vi "Main FPGA 8-axis_4.vi"() -> ()   [LabVIEW 2014]
uses:
  <vilib>/Motion/MotorControl/_s/nism.interpretControlRegister.stateTransition.ctl
  <vilib>/Platform/TimedLoop/XDataNode/timing_clust.ctl
  <vilib>/Platform/TimedLoop/XDataNode/nitl_modes.ctl
  <vilib>/Platform/TimedLoop/XDataNode/wakeup.ctl
  <vilib>/rvi/Emulation/niFpgaGetClockAttributes.vi
  <vilib>/rvi/Emulation/niFpgaSctlEmulationGetInTimedLoop.vi
  <vilib>/rvi/Emulation/niFpgaEmulationReportErrorSimple.vi
  Global FPGA 8-axis.vi
  <vilib>/rvi/eio/common/nirviEmuTemplateMethod_errors.vi
  <vilib>/Motion/MotorControl/_s/nism.interpretControlRegister.indexed.vi
  <vilib>/rvi/Emulation/niFpgaProcessEmulError.vi
  <vilib>/Motion/MotorControl/_s/nism.mdo.read.positionLoopSyncData.vi
  <vilib>/Motion/MotorControl/_s/nism.mdo.read.splineData.vi
  <vilib>/Motion/MotorControl/_s/nism.generateStatusRegister.indexed.vi
  <vilib>/rvi/Emulation/niFpgaCriticalErrorInLSC.vi
  <vilib>/Motion/MotorControl/_s/nism.splineInterpolation.fxp.3.index.vi
  <vilib>/Motion/MotorControl/_s/nism.mdo.handler.indexed.vi
  <vilib>/Motion/SoftMotion/Synchronization/nism.rioScan.generateSyncScan.vi
  <vilib>/eio/EIONode/EIONode.xnode
  <vilib>/Platform/TimedLoop/XDataNode/XDataNode.xnode
  <vilib>/Motion/MotorControl/NI_SoftMotion_MotorControlIP.lvlib
  <vilib>/Platform/TimedLoop/XDataNode/XDNodeRunTimeDep.lvlib
  <vilib>/Motion/SoftMotion/Synchronization/NI_SoftMotion_Synchronization.lvlib
panel:
  out "Interpolated Positions":fxp<+/-,64,32>[](array[numeric])
  in  "minimum pulse":u16=40
  in  "Invert direction?":bool
  in  "Enable Drives?":bool
  out "State":T1=enum."Start --> Initializing" caption="state transition"
  in  "Sync Value":bool
  in  "Sync Enable override?":bool
  out "Sync is Fault":bool
  out "Sync is Locked":bool
  # "Synchronization Loop"
  # "Control Status Loop"
  # "Notes: \n1. This VI provides the communication interface between the NI SoftMotion Engine and the LabVIEW FPGA Module. You must compile this VI for a specific FPGA target before use. After compiling, run the VI before running any of the Express VI examples. For information on moving this example to another FPGA target, refer to ni.com/info and enter info code fpgaex.\n\n2. Only use the Reset Axis button if you are unable to communicate with the axis by any other means. This button resets the device state machine and other VIs to a known state. After resetting the axis, switch the NI Scan Engine from Active Mode to Configuration Mode, then back to Active Mode, before attempting to enable the axis."
  # "(These two buttons \nare for testing\npurposes.)"
  # "Step/Direction Loop"
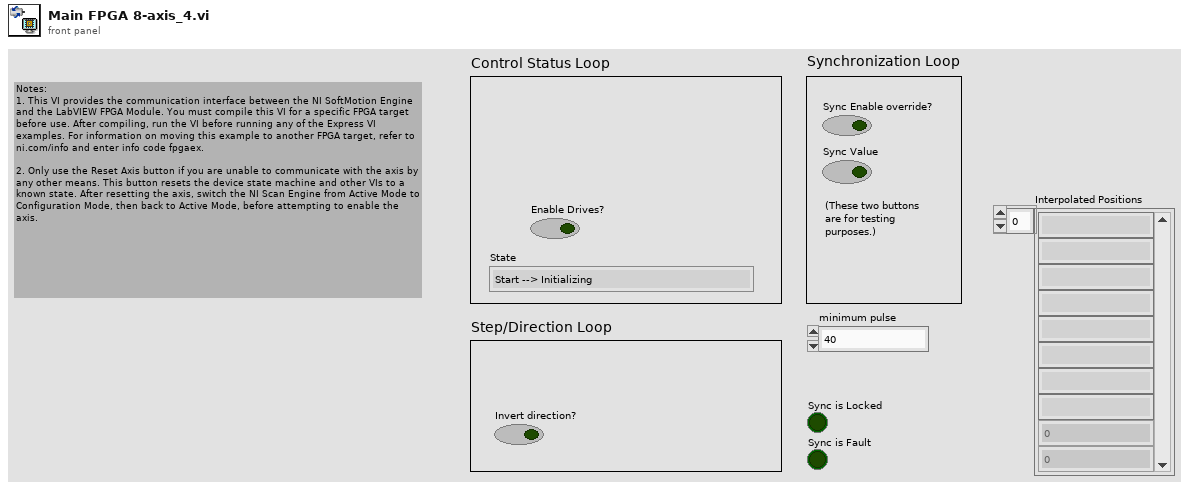
[diagram p1: front panel]
types:
  T1 = typedef "NI_SoftMotion_MotorControlIP.lvlib/nism.interpretControlRegister.stateTransition.ctl" = enum8{"Invalid", "Start --> Initializing", "Initializing --> Disabled", "Disabled --> Ready To Switch On", "Ready To Switch On --> Switched On", "Ready To Switch On --> Disable", "Switched On --> Operation Enable", "Switched On --> Ready To Switch On", "Switched On --> Disabled", "Operation Enable --> Switched On", "Operation Enable --> Ready To Switch On", "Operation Enable --> Disabled", "Fault --> Disabled", "Any --> Fault", "None"}
  T2 = typedef "NI_SoftMotion_MotorControlIP.lvlib/nism.mdo.splineData.ctl" = cluster{"spline type":T3, "traj per/spline per":u16, "spline per/traj per":fxp<+,32,0>}
  T3 = typedef "NI_SoftMotion_MotorControlIP.lvlib/nism.splineInterpolation.type.ctl" = u16
  T4 = typedef "NI_SoftMotion_Synchronization.lvlib/nism.softmotionScan.timerConfig.ctl" = cluster{"target period (clocks)":u16, "host period / target period":u16}
  T5 = typedef "NI_SoftMotion_Synchronization.lvlib/nism.softmotionScan.timerControl.ctl" = cluster{"sm scan":bool, "sm scan count":u32, "sm scan enabled":bool}
  T6 = typedef "XDNodeRunTimeDep.lvlib/timing_clust.ctl" = cluster{"Expected End [f-1]":u64, "Actual End [f-1]":u64, "Finished Late? [f-1]":bool, "Expected End [i-1]":u64, "Actual End [i-1]":u64, "Finished Late? [i-1]":bool, "Expected Start [i]":u64, "Actual Start [i]":u64, "Expected Start [f]":u64, "Actual Start [f]":u64, "Source Name":string, "Structure Name":string, "Period":i64, "Deadline":i64, "Offset":i64, "Start":i64, "Priority":i32, "Timeout":i32, "Mode":T7, "Wakeup Reason":T8, "Error":errorcluster, "Source Type":string, "Secondary Source Type":string, "Global End Time":u64, "Global Start Time":u64, "Frame Duration":u64, "Iteration Duration":u64, "Assigned CPU":i32, "I/O Scan Engine Mode":u32}
  T7 = typedef "XDNodeRunTimeDep.lvlib/nitl_modes.ctl" = enum32{"No Change", "Process missed periods, maintain original phase", "Discard missed periods, maintain original phase", "Process missed periods, ignore original phase", "Discard missed periods, ignore original phase"}
  T8 = typedef "XDNodeRunTimeDep.lvlib/wakeup.ctl" = enum32{"Normal", "Aborted", "Asynchronous wakeup", "Timing source error", "Timed loop error", "Timeout"}
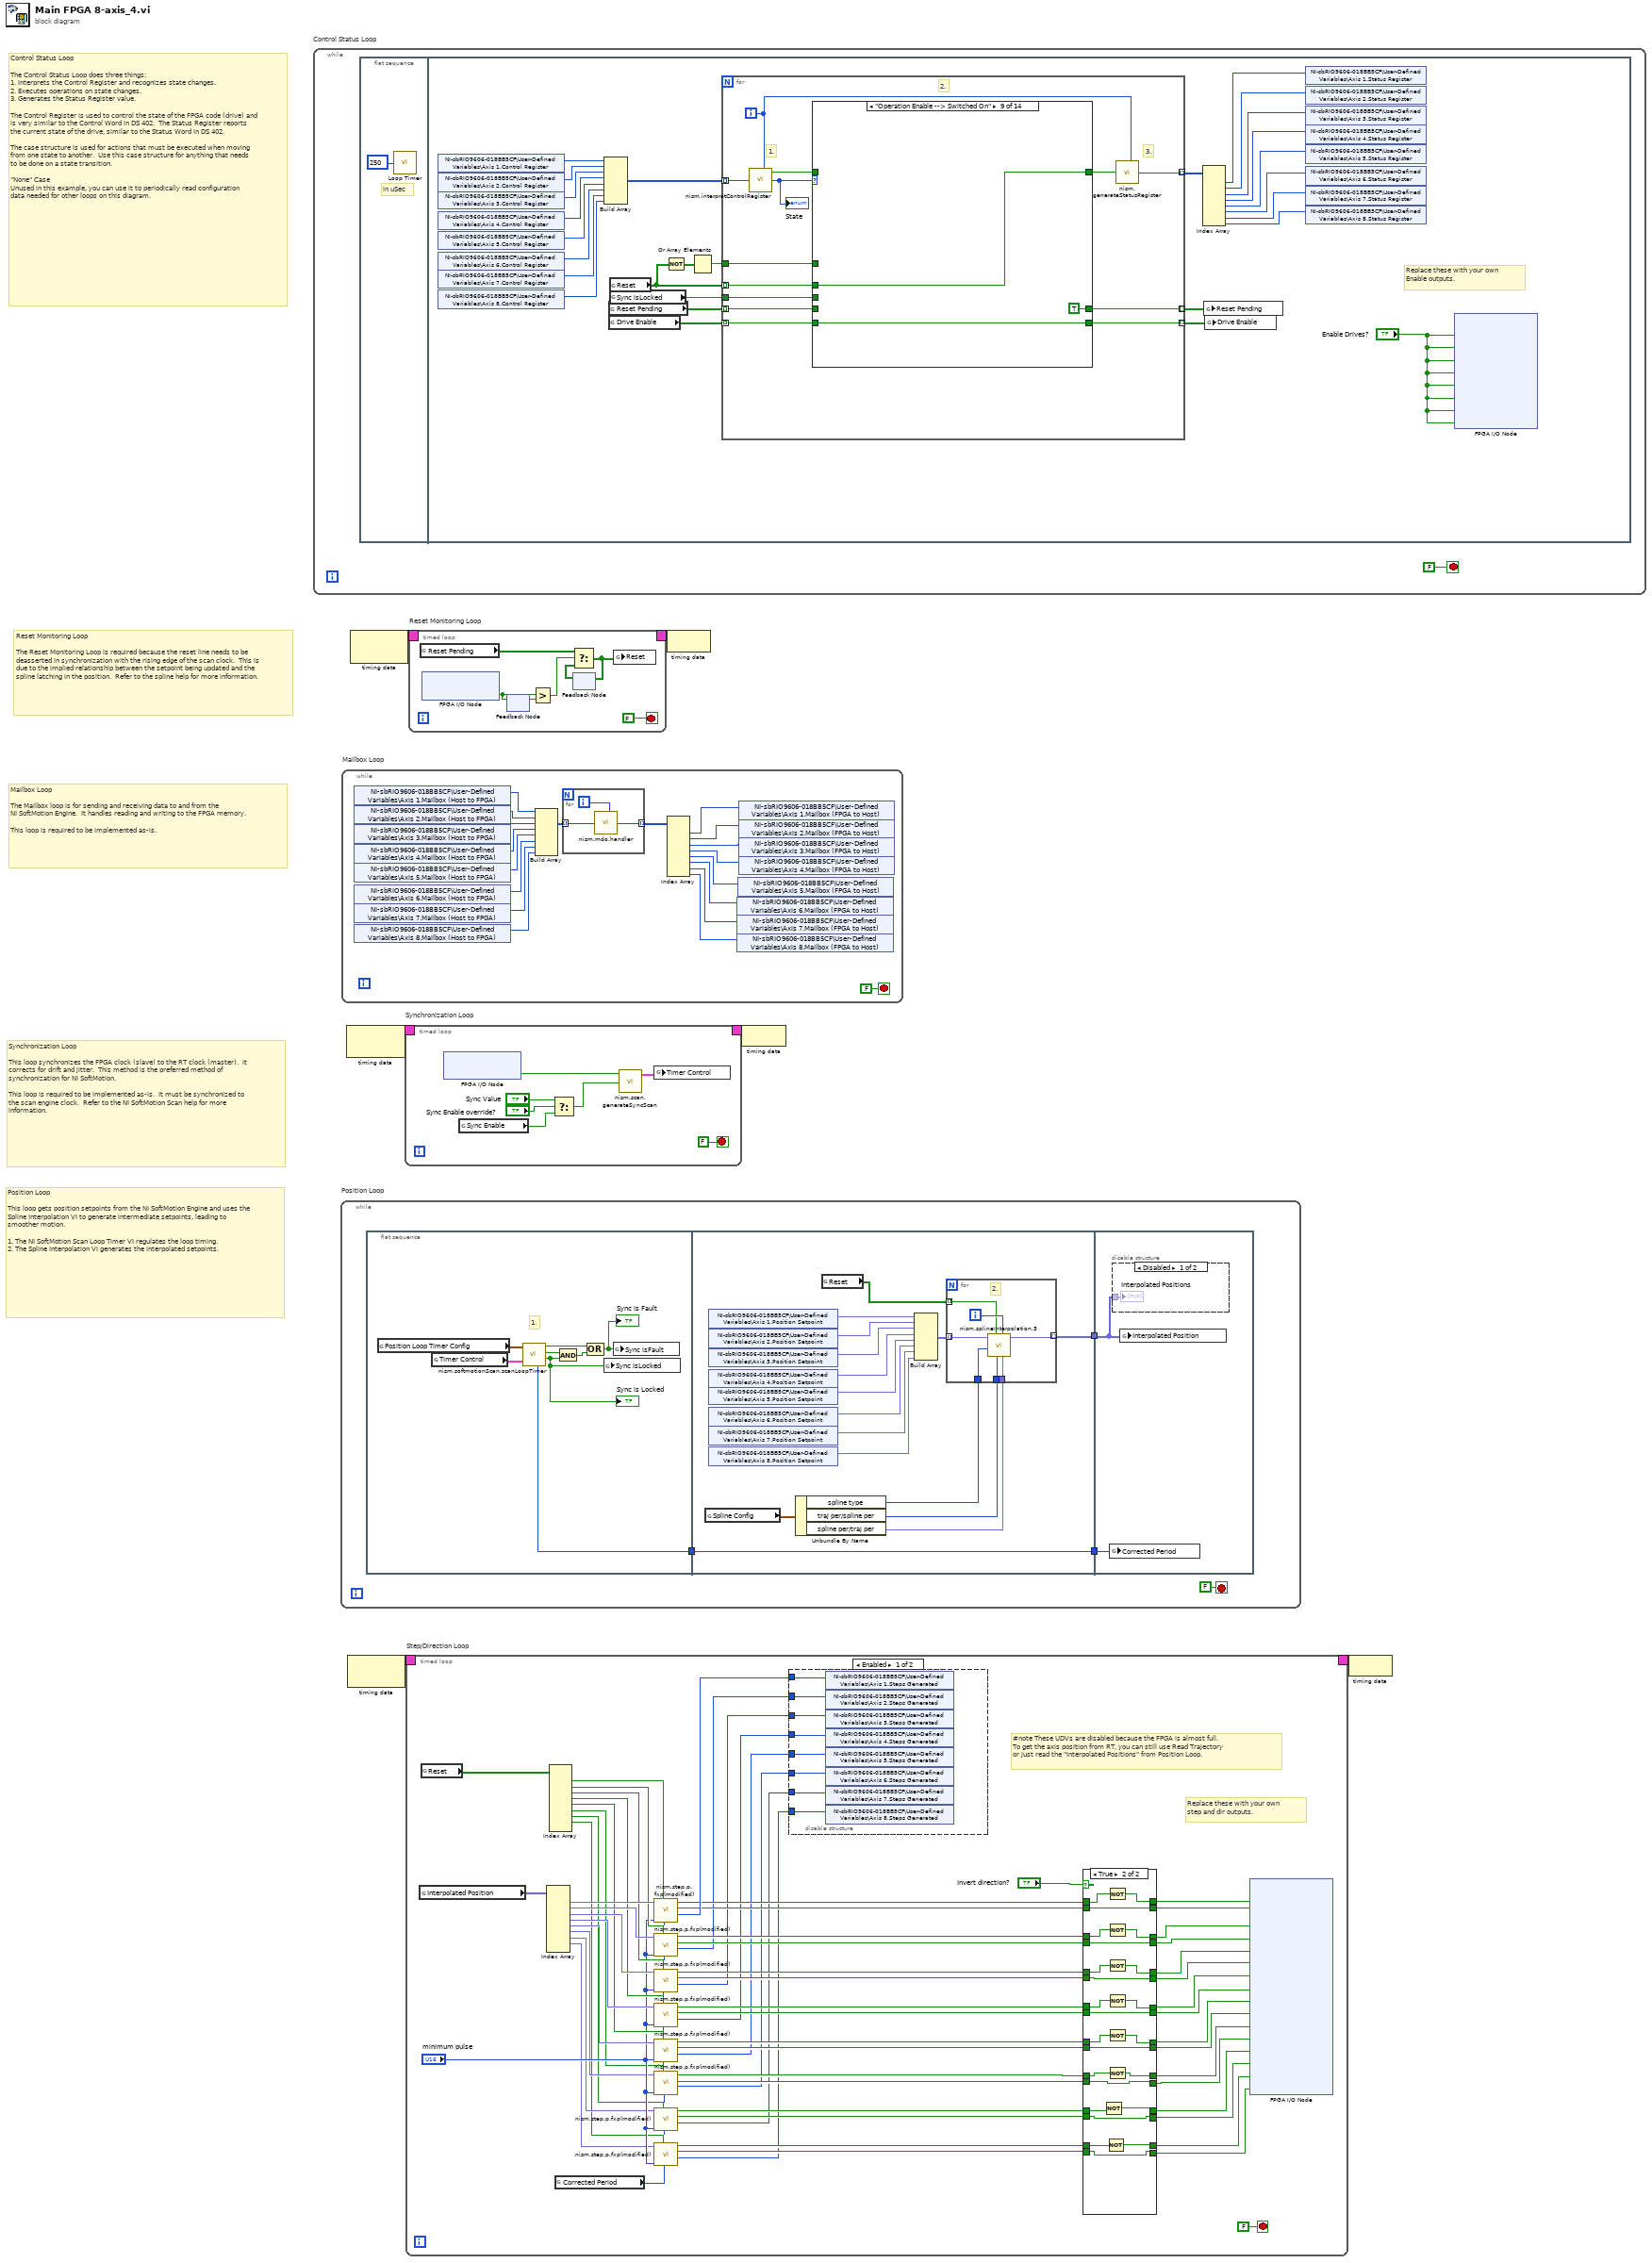
[diagram p0: block diagram]
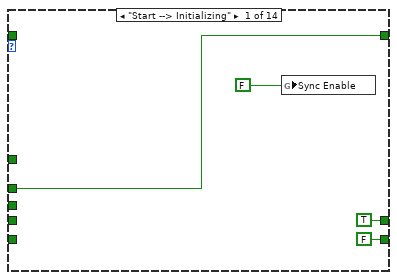
[diagram p5: hidden frame]
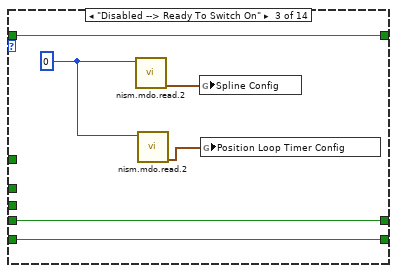
[diagram p7: hidden frame]
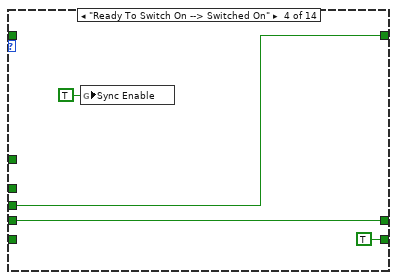
[diagram p8: hidden frame]
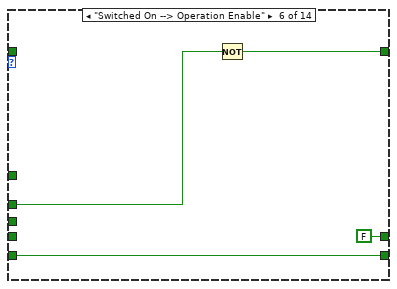
[diagram p10: hidden frame]
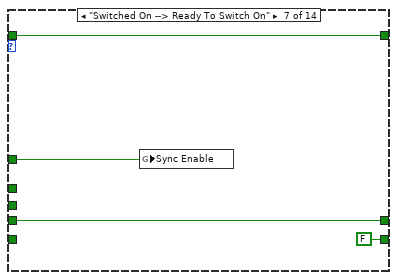
[diagram p11: hidden frame]
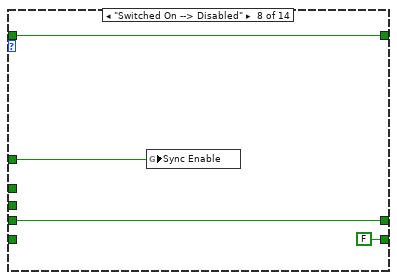
[diagram p12: hidden frame]
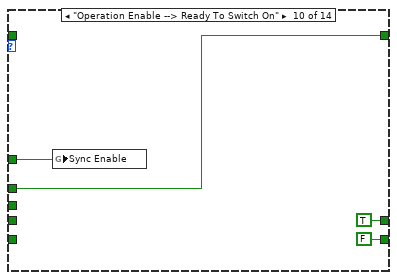
[diagram p13: hidden frame]
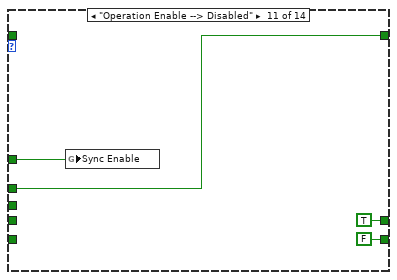
[diagram p14: hidden frame]
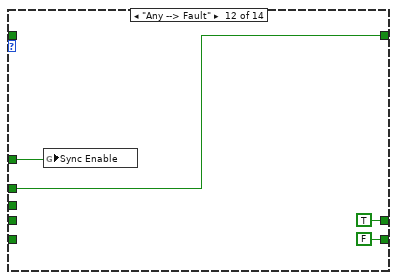
[diagram p15: hidden frame]
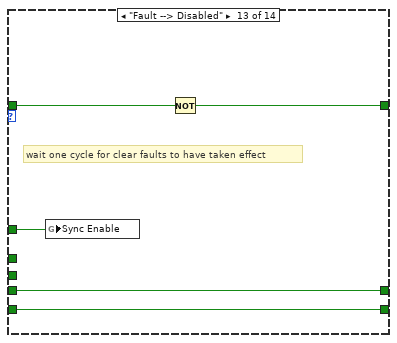
[diagram p16: hidden frame]
diagram:
  # "Position Loop\n\nThis loop gets position setpoints from the NI SoftMotion Engine and uses the Spline Interpolation VI to generate intermediate setpoints, leading to smoother motion.\n\n1. The NI SoftMotion Scan Loop Timer VI regulates the loop timing. \n2. The Spline Interpolation VI generates the interpolated setpoints."
  # "Synchronization Loop\n\nThis loop synchronizes the FPGA clock (slave) to the RT clock (master).  It corrects for drift and jitter.  This method is the preferred method of synchronization for NI SoftMotion.\n\nThis loop is required to be implemented as-is.  It must be synchronized to the scan engine clock.  Refer to the NI SoftMotion Scan help for more information."
  # "Mailbox Loop\n\nThe Mailbox loop is for sending and receiving data to and from the \nNI SoftMotion Engine.  It handles reading and writing to the FPGA memory.\n\nThis loop is required to be implemented as-is."
  # "Reset Monitoring Loop\n\nThe Reset Monitoring Loop is required because the reset line needs to be deasserted in synchronization with the rising edge of the scan clock.  This is due to the implied relationship between the setpoint being updated and the spline latching in the position.  Refer to the spline help for more information."
  # "Control Status Loop\n\nThe Control Status Loop does three things:\n1. Interprets the Control Register and recognizes state changes.\n2. Executes operations on state changes.\n3. Generates the Status Register value.\n\nThe Control Register is used to control the state of the FPGA code (drive) and is very similar to the Control Word in DS 402.  The Status Register reports the current state of the drive, similar to the Status Word in DS 402.\n\nThe case structure is used for actions that must be executed when moving from one state to another.  Use this case structure for anything that needs to be done on a state transition.\n\n\"None\" Case\nUnused in this example, you can use it to periodically read configuration data needed for other loops on this diagram."
  n1 = while "Control Status Loop" {
    stop <- FALSE stop-if-true
    n2 = flat-sequence {
      frame #0 {
        # "in uSec"
        n3 = call "Loop Timer"("Count(uSec)"=u32 250) -> ()  [unwired: 1 out]
      }
      frame #1 {
        # "Replace these with your own\nEnable outputs."
        n4 = shared-variable "NI-sbRIO9606-018BB5CF\\User-Defined Variables\\Axis 1.Control Register"() -> (w25:u32)  [unwired: 1 in, 1 out]
        n5 = shared-variable "NI-sbRIO9606-018BB5CF\\User-Defined Variables\\Axis 2.Control Register"() -> (w24:u32)  [unwired: 1 in, 1 out]
        n6 = shared-variable "NI-sbRIO9606-018BB5CF\\User-Defined Variables\\Axis 3.Control Register"() -> (w23:u32)  [unwired: 1 in, 1 out]
        n7 = shared-variable "NI-sbRIO9606-018BB5CF\\User-Defined Variables\\Axis 4.Control Register"() -> (w22:u32)  [unwired: 1 in, 1 out]
        n8 = shared-variable "NI-sbRIO9606-018BB5CF\\User-Defined Variables\\Axis 5.Control Register"() -> (w21:u32)  [unwired: 1 in, 1 out]
        n9 = shared-variable "NI-sbRIO9606-018BB5CF\\User-Defined Variables\\Axis 6.Control Register"() -> (w15:u32)  [unwired: 1 in, 1 out]
        n10 = shared-variable "NI-sbRIO9606-018BB5CF\\User-Defined Variables\\Axis 7.Control Register"() -> (w14:u32)  [unwired: 1 in, 1 out]
        n11 = shared-variable "NI-sbRIO9606-018BB5CF\\User-Defined Variables\\Axis 8.Control Register"() -> (w13:u32)  [unwired: 1 in, 1 out]
        n12 = Build Array(w25, w24, w23, w22, w21, w15, w14, w13) -> (w34:u32[])
        n13 = global read "Global FPGA 8-axis.vi" "Reset Pending"() -> (w29:bool[])
        n14 = global read "Global FPGA 8-axis.vi" "Drive Enable"() -> (w28:bool[])
        n15 = global read "Global FPGA 8-axis.vi" "Reset"() -> (w30:bool[])
        n16 = global read "Global FPGA 8-axis.vi" "Sync isLocked"() -> (w35:bool)
        n17 = Not(x=w30) -> (.not. x?=w32:bool[])
        n18 = Or Array Elements(Boolean array=w32) -> (logical OR=w31:bool)
        n19 = for {
          tunnel: w30 -> [w43] mode=indexing
          tunnel: w35 -> [w42]
          tunnel: w34 -> [w44] mode=indexing
          tunnel: [w41] -> w26 mode=indexing
          tunnel: [w40] -> w33 mode=indexing
          tunnel: [w39] -> w27 mode=indexing
          tunnel: w31 -> [w38]
          tunnel: w29 -> [w37] mode=indexing
          tunnel: w28 -> [w36] mode=indexing
          i -> [w45]
          # "3."
          # "2."
          # "1."
          n20 = call-poly <vilib>:"nism.interpretControlRegister.vi"("control register"=w44, "axis index"=w45) -> ("transition occurred"=w46:bool, "state transition"=w47:T1)  [unwired: 6 in]
          "State" <- w47
          n21 = case shown="\"Operation Enable --> Switched On\"" w47 {
            tunnel: w46 -> [_ w55 w61 _ w68 _ w76 w80 _ _ _ _ w100 _]
            tunnel: [w52 w55 w61 w63 w68 w72 w76 w80 w82 w85 w89 w93 w99 _] -> w48
            tunnel: w43 -> [w52 _ _ _ _ w71 _ _ w82 w85 w89 w93 _ _]
            tunnel: w42 -> [_ _ _ w63 _ _ _ _ _ _ _ _ _ _]
            tunnel: [TRUE ("Write.Reset Pending") w54 w57 w62 w67 FALSE ("Write.Reset Pending") w73 w77 TRUE ("Write.Reset Pending") TRUE ("Write.Reset Pending") TRUE ("Write.Reset Pending") TRUE ("Write.Reset Pending") w97 w102] -> w40
            tunnel: [FALSE ("Write.Drive Enable") w53 w56 TRUE ("Write.Drive Enable") w66 w69 FALSE ("Write.Drive Enable") FALSE ("Write.Drive Enable") w81 FALSE ("Write.Drive Enable") FALSE ("Write.Drive Enable") FALSE ("Write.Drive Enable") w96 w101] -> w39
            tunnel: w38 -> [_ _ _ _ _ _ w74 w78 _ w84 w88 w92 w98 _]
            tunnel: w37 -> [_ w54 w57 w62 w67 _ w73 w77 _ _ _ _ w97 w102]
            tunnel: w36 -> [_ w53 w56 _ w66 w69 _ _ w81 _ _ _ w96 w101]
            frame "Start --> Initializing" {
              n22 = global write "Global FPGA 8-axis.vi" "Sync Enable"(FALSE ("Sync Enable")) -> ()
            }
            frame "Initializing --> Disabled" {
            }
            frame "Disabled --> Ready To Switch On" {
              w59 = 0 ("axis index")
              n23 = call-poly <vilib>:"nism.mdo.read.2.vi"("axis index"=w59) -> ("spline"=w60:T2)  [unwired: 10 in]
              n24 = call-poly <vilib>:"nism.mdo.read.2.vi"("axis index"=w59) -> ("position loop sync"=w58:T4)  [unwired: 10 in]
              n25 = global write "Global FPGA 8-axis.vi" "Spline Config"(w60) -> ()
              n26 = global write "Global FPGA 8-axis.vi" "Position Loop Timer Config"(w58) -> ()
            }
            frame "Ready To Switch On --> Switched On" {
              n27 = global write "Global FPGA 8-axis.vi" "Sync Enable"(TRUE ("Sync Enable")) -> ()
            }
            frame "Ready To Switch On --> Disable" {
            }
            frame "Switched On --> Operation Enable" {
              n28 = Not(x=w71) -> (.not. x?=w72:bool)
            }
            frame "Switched On --> Ready To Switch On" {
              n29 = global write "Global FPGA 8-axis.vi" "Sync Enable"(w74) -> ()
            }
            frame "Switched On --> Disabled" {
              n30 = global write "Global FPGA 8-axis.vi" "Sync Enable"(w78) -> ()
            }
            frame "Operation Enable --> Switched On" {
            }
            frame "Operation Enable --> Ready To Switch On" {
              n31 = global write "Global FPGA 8-axis.vi" "Sync Enable"(w84) -> ()
            }
            frame "Operation Enable --> Disabled" {
              n32 = global write "Global FPGA 8-axis.vi" "Sync Enable"(w88) -> ()
            }
            frame "Any --> Fault" {
              n33 = global write "Global FPGA 8-axis.vi" "Sync Enable"(w92) -> ()
            }
            frame "Fault --> Disabled" {
              # "wait one cycle for clear faults to have taken effect"
              n34 = global write "Global FPGA 8-axis.vi" "Sync Enable"(w98) -> ()
              n35 = Not(x=w100) -> (.not. x?=w99:bool)
            }
            frame "None", Default {
            }
          }
          n36 = call-poly <vilib>:"nism.generateStatusRegister.vi"("transition success"=w48, "axis index"=w45) -> ("status register"=w41:u32)  [unwired: 7 in]
        }
        n37 = Index Array(array=w26) -> (element #1=w20:u32, element #2=w19:u32, element #3=w18:u32, element #4=w17:u32, element #5=w16:u32, element #6=w12:u32, element #7=w11:u32, element #8=w10:u32)  [unwired: 8 in]
        n38 = global write "Global FPGA 8-axis.vi" "Reset Pending"(w33) -> ()
        n39 = global write "Global FPGA 8-axis.vi" "Drive Enable"(w27) -> ()
        n40 = shared-variable "NI-sbRIO9606-018BB5CF\\User-Defined Variables\\Axis 1.Status Register"(w20) -> ()  [unwired: 1 in, 1 out]
        n41 = shared-variable "NI-sbRIO9606-018BB5CF\\User-Defined Variables\\Axis 2.Status Register"(w19) -> ()  [unwired: 1 in, 1 out]
        n42 = shared-variable "NI-sbRIO9606-018BB5CF\\User-Defined Variables\\Axis 3.Status Register"(w18) -> ()  [unwired: 1 in, 1 out]
        n43 = shared-variable "NI-sbRIO9606-018BB5CF\\User-Defined Variables\\Axis 4.Status Register"(w17) -> ()  [unwired: 1 in, 1 out]
        n44 = shared-variable "NI-sbRIO9606-018BB5CF\\User-Defined Variables\\Axis 5.Status Register"(w16) -> ()  [unwired: 1 in, 1 out]
        n45 = shared-variable "NI-sbRIO9606-018BB5CF\\User-Defined Variables\\Axis 6.Status Register"(w12) -> ()  [unwired: 1 in, 1 out]
        n46 = shared-variable "NI-sbRIO9606-018BB5CF\\User-Defined Variables\\Axis 7.Status Register"(w11) -> ()  [unwired: 1 in, 1 out]
        n47 = shared-variable "NI-sbRIO9606-018BB5CF\\User-Defined Variables\\Axis 8.Status Register"(w10) -> ()  [unwired: 1 in, 1 out]
        n48 = xnode "FPGA I/O Node"("RMC/DIO15"="Enable Drives?", "RMC/DIO79"="Enable Drives?", "RMC/DIO78"="Enable Drives?", "RMC/DIO13"="Enable Drives?", "RMC/DIO62"="Enable Drives?", "RMC/DIO61"="Enable Drives?", "RMC/DIO76"="Enable Drives?", "RMC/DIO11"="Enable Drives?") -> ()  [unwired: 8 in, 8 out]
      }
    }
  }
  n49 = while "Position Loop" {
    stop <- FALSE stop-if-true
    n50 = flat-sequence {
      tunnel: [w107] -> w103
      tunnel: [w124] -> w105
      tunnel: [w123] -> w104
      tunnel: w103 -> [w123]
      tunnel: w105 -> [w138]
      tunnel: w104 -> [w139]
      frame #0 {
        # "1."
        n51 = global read "Global FPGA 8-axis.vi" "Position Loop Timer Config"() -> (w109:T4)
        n52 = global read "Global FPGA 8-axis.vi" "Timer Control"() -> (w108:T5)
        n53 = call <vilib>:"nism.softmotionScan.scanLoopTimer.vi"("timer control"=w108, "timer config"=w109) -> ("scan running?"=w111:bool, "finished late?"=w113:bool, "fault occurred?"=w114:bool, "corrected period"=w107:u16)  [unwired: 5 in, 1 out]
        "Sync is Locked" <- w111
        n54 = Compound Arithmetic op=AND(w113, w111) -> (w112:bool)
        n55 = Compound Arithmetic op=OR(w114, w112) -> (w110:bool)
        "Sync is Fault" <- w110
        n56 = global write "Global FPGA 8-axis.vi" "Sync isLocked"(w111) -> ()
        n57 = global write "Global FPGA 8-axis.vi" "Sync isFault"(w110) -> ()
      }
      frame #1 {
        n58 = global read "Global FPGA 8-axis.vi" "Spline Config"() -> (w126:T2)
        n59 = shared-variable "NI-sbRIO9606-018BB5CF\\User-Defined Variables\\Axis 1.Position Setpoint"() -> (w122:fxp<+/-,64,32>)  [unwired: 1 in, 1 out]
        n60 = shared-variable "NI-sbRIO9606-018BB5CF\\User-Defined Variables\\Axis 2.Position Setpoint"() -> (w121:fxp<+/-,64,32>)  [unwired: 1 in, 1 out]
        n61 = shared-variable "NI-sbRIO9606-018BB5CF\\User-Defined Variables\\Axis 3.Position Setpoint"() -> (w120:fxp<+/-,64,32>)  [unwired: 1 in, 1 out]
        n62 = shared-variable "NI-sbRIO9606-018BB5CF\\User-Defined Variables\\Axis 4.Position Setpoint"() -> (w119:fxp<+/-,64,32>)  [unwired: 1 in, 1 out]
        n63 = shared-variable "NI-sbRIO9606-018BB5CF\\User-Defined Variables\\Axis 5.Position Setpoint"() -> (w118:fxp<+/-,64,32>)  [unwired: 1 in, 1 out]
        n64 = shared-variable "NI-sbRIO9606-018BB5CF\\User-Defined Variables\\Axis 6.Position Setpoint"() -> (w117:fxp<+/-,64,32>)  [unwired: 1 in, 1 out]
        n65 = shared-variable "NI-sbRIO9606-018BB5CF\\User-Defined Variables\\Axis 7.Position Setpoint"() -> (w116:fxp<+/-,64,32>)  [unwired: 1 in, 1 out]
        n66 = shared-variable "NI-sbRIO9606-018BB5CF\\User-Defined Variables\\Axis 8.Position Setpoint"() -> (w115:fxp<+/-,64,32>)  [unwired: 1 in, 1 out]
        n67 = Unbundle By Name(w126) -> ("spline type"=w130:T3, "traj per/spline per"=w129:u16, "spline per/traj per"=w128:fxp<+,32,0>)
        n68 = global read "Global FPGA 8-axis.vi" "Reset"() -> (w125:bool[])
        n69 = Build Array(w122, w121, w120, w119, w118, w117, w116, w115) -> (w127:fxp<+/-,64,32>[])
        n70 = for {
          tunnel: w130 -> [w137]
          tunnel: w129 -> [w136]
          tunnel: w128 -> [w135]
          tunnel: w125 -> [w132] mode=indexing
          tunnel: w127 -> [w134] mode=indexing
          tunnel: [w131] -> w124 mode=indexing
          i -> [w133]
          # "2."
          n71 = call-poly <vilib>:"nism.splineInterpolation.3.vi"("1 / calls per sample"=w135, "index"=w133, "calls per sample"=w136, "reset"=w132, "spline type"=w137, "x"=w134) -> ("xi"=w131:fxp<+/-,64,32>)  [unwired: 4 in, 1 out]
        }
      }
      frame #2 {
        n72 = global write "Global FPGA 8-axis.vi" "Corrected Period"(w139) -> ()
        n73 = disable-structure shown="Disabled" {
          disable-tunnel: w138 -> [w140 _]
          frame Disabled {
            "Interpolated Positions" <- w140
          }
          frame Enabled {
          }
        }
        n74 = global write "Global FPGA 8-axis.vi" "Interpolated Position"(w138) -> ()
      }
    }
  }
  n75 = while "Mailbox Loop" {
    stop <- FALSE stop-if-true
    n76 = shared-variable "NI-sbRIO9606-018BB5CF\\User-Defined Variables\\Axis 1.Mailbox (Host to FPGA)"() -> (w156:u64)  [unwired: 1 in, 1 out]
    n77 = shared-variable "NI-sbRIO9606-018BB5CF\\User-Defined Variables\\Axis 2.Mailbox (Host to FPGA)"() -> (w155:u64)  [unwired: 1 in, 1 out]
    n78 = shared-variable "NI-sbRIO9606-018BB5CF\\User-Defined Variables\\Axis 3.Mailbox (Host to FPGA)"() -> (w154:u64)  [unwired: 1 in, 1 out]
    n79 = shared-variable "NI-sbRIO9606-018BB5CF\\User-Defined Variables\\Axis 4.Mailbox (Host to FPGA)"() -> (w153:u64)  [unwired: 1 in, 1 out]
    n80 = shared-variable "NI-sbRIO9606-018BB5CF\\User-Defined Variables\\Axis 5.Mailbox (Host to FPGA)"() -> (w152:u64)  [unwired: 1 in, 1 out]
    n81 = shared-variable "NI-sbRIO9606-018BB5CF\\User-Defined Variables\\Axis 6.Mailbox (Host to FPGA)"() -> (w146:u64)  [unwired: 1 in, 1 out]
    n82 = shared-variable "NI-sbRIO9606-018BB5CF\\User-Defined Variables\\Axis 7.Mailbox (Host to FPGA)"() -> (w145:u64)  [unwired: 1 in, 1 out]
    n83 = shared-variable "NI-sbRIO9606-018BB5CF\\User-Defined Variables\\Axis 8.Mailbox (Host to FPGA)"() -> (w144:u64)  [unwired: 1 in, 1 out]
    n84 = Build Array(w156, w155, w154, w153, w152, w146, w145, w144) -> (w158:u64[])
    n85 = for {
      tunnel: w158 -> [w162] mode=indexing
      tunnel: [w161] -> w157 mode=indexing
      i -> [w160]
      n86 = call-poly <vilib>:"nism.mdo.handler.vi"("mbox (host to fpga)"=w162, "axis index"=w160) -> ("mbox (fpga to host)"=w161:u64)  [unwired: 7 in]
    }
    n87 = Index Array(array=w157) -> (element #1=w151:u64, element #2=w150:u64, element #3=w149:u64, element #4=w148:u64, element #5=w147:u64, element #6=w143:u64, element #7=w142:u64, element #8=w141:u64)  [unwired: 8 in]
    n88 = shared-variable "NI-sbRIO9606-018BB5CF\\User-Defined Variables\\Axis 6.Mailbox (FPGA to Host)"(w143) -> ()  [unwired: 1 in, 1 out]
    n89 = shared-variable "NI-sbRIO9606-018BB5CF\\User-Defined Variables\\Axis 7.Mailbox (FPGA to Host)"(w142) -> ()  [unwired: 1 in, 1 out]
    n90 = shared-variable "NI-sbRIO9606-018BB5CF\\User-Defined Variables\\Axis 8.Mailbox (FPGA to Host)"(w141) -> ()  [unwired: 1 in, 1 out]
    n91 = shared-variable "NI-sbRIO9606-018BB5CF\\User-Defined Variables\\Axis 5.Mailbox (FPGA to Host)"(w147) -> ()  [unwired: 1 in, 1 out]
    n92 = shared-variable "NI-sbRIO9606-018BB5CF\\User-Defined Variables\\Axis 1.Mailbox (FPGA to Host)"(w151) -> ()  [unwired: 1 in, 1 out]
    n93 = shared-variable "NI-sbRIO9606-018BB5CF\\User-Defined Variables\\Axis 2.Mailbox (FPGA to Host)"(w150) -> ()  [unwired: 1 in, 1 out]
    n94 = shared-variable "NI-sbRIO9606-018BB5CF\\User-Defined Variables\\Axis 3.Mailbox (FPGA to Host)"(w149) -> ()  [unwired: 1 in, 1 out]
    n95 = shared-variable "NI-sbRIO9606-018BB5CF\\User-Defined Variables\\Axis 4.Mailbox (FPGA to Host)"(w148) -> ()  [unwired: 1 in, 1 out]
  }
  n96 = node-c288() -> (w6:T6)  [unwired: 1 in]
  n97 = node-c288() -> (w2:T6)  [unwired: 1 in]
  n98 = node-c288() -> (w4:T6)  [unwired: 1 in]
  n99 = timed-loop "Synchronization Loop" {
    timing: w6 -> [_]
    timing-out: [_] -> w5
    stop <- FALSE stop-if-true
    n100 = xnode "FPGA I/O Node"() -> ("Scan Clock"=w167:bool)  [unwired: 1 in, 1 out]
    n101 = global read "Global FPGA 8-axis.vi" "Sync Enable"() -> (w166:bool)
    n102 = Select(t="Sync Value", s="Sync Enable override?", f=w166) -> (s? t:f=w163:bool)
    n103 = call-poly <vilib>:"nism.scan.generateSyncScan.vi"("scan enable?"=w163, "scan clock"=w167) -> ("timer control"=w168:T5)  [unwired: 3 in]
    n104 = global write "Global FPGA 8-axis.vi" "Timer Control"(w168) -> ()
  }
  n105 = timed-loop "Step/Direction Loop" {
    timing: w2 -> [_]
    timing-out: [_] -> w1
    stop <- FALSE stop-if-true
    # "#note These UDVs are disabled because the FPGA is almost full.\nTo get the axis position from RT, you can still use Read Trajectory\nor just read the \"Interpolated Positions\" from Position Loop."
    # "Replace these with your own\nstep and dir outputs."
    n106 = global read "Global FPGA 8-axis.vi" "Interpolated Position"() -> (w232:fxp<+/-,64,32>[])
    n107 = global read "Global FPGA 8-axis.vi" "Reset"() -> (w226:bool[])
    n108 = Index Array(array=w232) -> (element #1=w231:fxp<+/-,64,32>, element #2=w230:fxp<+/-,64,32>, element #3=w229:fxp<+/-,64,32>, element #4=w228:fxp<+/-,64,32>, element #5=w227:fxp<+/-,64,32>, element #6=w194:fxp<+/-,64,32>, element #7=w193:fxp<+/-,64,32>, element #8=w192:fxp<+/-,64,32>)  [unwired: 9 in, 1 out]
    n109 = Index Array(array=w226) -> (element #1=w225:bool, element #2=w224:bool, element #3=w223:bool, element #4=w222:bool, element #5=w221:bool, element #6=w191:bool, element #7=w190:bool, element #8=w189:bool)  [unwired: 9 in, 1 out]
    n110 = global read "Global FPGA 8-axis.vi" "Corrected Period"() -> (w182:u16)
    n111 = call "nism.step.p.fxp(modified).vi"("calls per sample"=w182, "reset"=w225, "minimum pulse"="minimum pulse", "position setpoint"=w231) -> ("steps generated"=w220:i32, "step"=w218:bool, "direction"=w219:bool)  [unwired: 4 in, 1 out]
    n112 = call "nism.step.p.fxp(modified).vi"("calls per sample"=w182, "reset"=w224, "minimum pulse"="minimum pulse", "position setpoint"=w230) -> ("steps generated"=w209:i32, "step"=w216:bool, "direction"=w217:bool)  [unwired: 4 in, 1 out]
    n113 = call "nism.step.p.fxp(modified).vi"("calls per sample"=w182, "reset"=w223, "minimum pulse"="minimum pulse", "position setpoint"=w229) -> ("steps generated"=w208:i32, "step"=w214:bool, "direction"=w215:bool)  [unwired: 4 in, 1 out]
    n114 = call "nism.step.p.fxp(modified).vi"("calls per sample"=w182, "reset"=w222, "minimum pulse"="minimum pulse", "position setpoint"=w228) -> ("steps generated"=w207:i32, "step"=w212:bool, "direction"=w213:bool)  [unwired: 4 in, 1 out]
    n115 = call "nism.step.p.fxp(modified).vi"("calls per sample"=w182, "reset"=w221, "minimum pulse"="minimum pulse", "position setpoint"=w227) -> ("steps generated"=w206:i32, "step"=w210:bool, "direction"=w211:bool)  [unwired: 4 in, 1 out]
    n116 = call "nism.step.p.fxp(modified).vi"("calls per sample"=w182, "reset"=w191, "minimum pulse"="minimum pulse", "position setpoint"=w194) -> ("steps generated"=w197:i32, "step"=w203:bool, "direction"=w204:bool)  [unwired: 4 in, 1 out]
    n117 = call "nism.step.p.fxp(modified).vi"("calls per sample"=w182, "reset"=w190, "minimum pulse"="minimum pulse", "position setpoint"=w193) -> ("steps generated"=w196:i32, "step"=w201:bool, "direction"=w202:bool)  [unwired: 4 in, 1 out]
    n118 = call "nism.step.p.fxp(modified).vi"("calls per sample"=w182, "reset"=w189, "minimum pulse"="minimum pulse", "position setpoint"=w192) -> ("steps generated"=w195:i32, "step"=w199:bool, "direction"=w200:bool)  [unwired: 4 in, 1 out]
    n119 = disable-structure shown="Enabled" {
      disable-tunnel: w220 -> [w241 _]
      disable-tunnel: w209 -> [w240 _]
      disable-tunnel: w208 -> [w239 _]
      disable-tunnel: w207 -> [w238 _]
      disable-tunnel: w206 -> [w237 _]
      disable-tunnel: w197 -> [w236 _]
      disable-tunnel: w196 -> [w235 _]
      disable-tunnel: w195 -> [w234 _]
      frame Enabled {
        n120 = shared-variable "NI-sbRIO9606-018BB5CF\\User-Defined Variables\\Axis 1.Steps Generated"(w241) -> ()  [unwired: 1 in, 1 out]
        n121 = shared-variable "NI-sbRIO9606-018BB5CF\\User-Defined Variables\\Axis 2.Steps Generated"(w240) -> ()  [unwired: 1 in, 1 out]
        n122 = shared-variable "NI-sbRIO9606-018BB5CF\\User-Defined Variables\\Axis 3.Steps Generated"(w239) -> ()  [unwired: 1 in, 1 out]
        n123 = shared-variable "NI-sbRIO9606-018BB5CF\\User-Defined Variables\\Axis 4.Steps Generated"(w238) -> ()  [unwired: 1 in, 1 out]
        n124 = shared-variable "NI-sbRIO9606-018BB5CF\\User-Defined Variables\\Axis 5.Steps Generated"(w237) -> ()  [unwired: 1 in, 1 out]
        n125 = shared-variable "NI-sbRIO9606-018BB5CF\\User-Defined Variables\\Axis 6.Steps Generated"(w236) -> ()  [unwired: 1 in, 1 out]
        n126 = shared-variable "NI-sbRIO9606-018BB5CF\\User-Defined Variables\\Axis 7.Steps Generated"(w235) -> ()  [unwired: 1 in, 1 out]
        n127 = shared-variable "NI-sbRIO9606-018BB5CF\\User-Defined Variables\\Axis 8.Steps Generated"(w234) -> ()  [unwired: 1 in, 1 out]
      }
      frame Disabled {
      }
    }
    n128 = case shown="True" "Invert direction?" {
      tunnel: w219 -> [w257 w281]
      tunnel: [w257 w280] -> w181
      tunnel: w217 -> [w255 w279]
      tunnel: [w255 w278] -> w179
      tunnel: w215 -> [w253 w277]
      tunnel: [w253 w276] -> w177
      tunnel: w213 -> [w251 w275]
      tunnel: [w251 w274] -> w175
      tunnel: w211 -> [w249 w273]
      tunnel: [w249 w272] -> w173
      tunnel: w218 -> [w256 w271]
      tunnel: [w256 w271] -> w180
      tunnel: w216 -> [w254 w270]
      tunnel: [w254 w270] -> w178
      tunnel: w214 -> [w252 w269]
      tunnel: [w252 w269] -> w176
      tunnel: w212 -> [w250 w268]
      tunnel: [w250 w268] -> w174
      tunnel: w210 -> [w248 w267]
      tunnel: [w248 w267] -> w172
      tunnel: w204 -> [w247 w266]
      tunnel: w203 -> [w246 w259]
      tunnel: w202 -> [w245 w265]
      tunnel: w201 -> [w244 w261]
      tunnel: w200 -> [w243 w264]
      tunnel: w199 -> [w242 w262]
      tunnel: [w247 w258] -> w188
      tunnel: [w246 w259] -> w187
      tunnel: [w245 w260] -> w186
      tunnel: [w244 w261] -> w185
      tunnel: [w243 w263] -> w184
      tunnel: [w242 w262] -> w183
      frame False {
      }
      frame True {
        n129 = Not(x=w265) -> (.not. x?=w260:bool)
        n130 = Not(x=w264) -> (.not. x?=w263:bool)
        n131 = Not(x=w281) -> (.not. x?=w280:bool)
        n132 = Not(x=w279) -> (.not. x?=w278:bool)
        n133 = Not(x=w277) -> (.not. x?=w276:bool)
        n134 = Not(x=w275) -> (.not. x?=w274:bool)
        n135 = Not(x=w273) -> (.not. x?=w272:bool)
        n136 = Not(x=w266) -> (.not. x?=w258:bool)
      }
    }
    n137 = xnode "FPGA I/O Node"("RMC/DIO46"=w181, "RMC/DIO47"=w180, "RMC/DIO14"=w179, "RMC/DIO63"=w178, "RMC/DIO95"=w177, "RMC/DIO31"=w176, "RMC/DIO30"=w175, "RMC/DIO45"=w174, "RMC/DIO77"=w173, "RMC/DIO44"=w172, "RMC/DIO12"=w188, "RMC/DIO94"=w187, "RMC/DIO93"=w186, "RMC/DIO29"=w185, "RMC/DIO28"=w184, "RMC/DIO43"=w183) -> ()  [unwired: 16 in, 16 out]
  }
  n138 = timed-loop "Reset Monitoring Loop" {
    timing: w4 -> [_]
    timing-out: [_] -> w3
    stop <- FALSE stop-if-true
    n139 = global read "Global FPGA 8-axis.vi" "Reset Pending"() -> (w286:bool[])
    n140 = xnode "FPGA I/O Node"() -> ("Scan Clock"=w285:bool)  [unwired: 1 in, 1 out]
    n141 = feedback-in #1(w285) -> ()
    n142 = feedback #1() -> (w284:bool)  [unwired: 1 in]
    n143 = Greater?(x=w285, y=w284) -> (0:w290:bool)
    n144 = feedback #2() -> (w289:bool[])  [unwired: 1 in]
    n145 = Select(t=w286, s=w290, f=w289) -> (s? t:f=w287:bool[])
    n146 = feedback-in #2(w287) -> ()
    n147 = global write "Global FPGA 8-axis.vi" "Reset"(w287) -> ()
  }
  n148 = node-c288(w3) -> ()
  n149 = node-c288(w5) -> ()
  n150 = node-c288(w1) -> ()
